vi "Get Sizes.vi"(2 "Array":variant) -> (0 "Sizes(s)":i32[](array[numeric]))   [LabVIEW 2019, in "Arrays.lvlib"]
uses:
  Arrays.lvlib
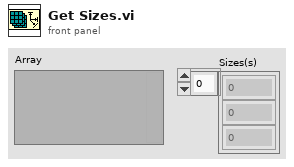
[diagram p1: front panel]
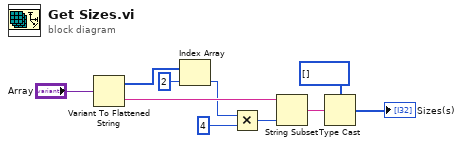
[diagram p0: block diagram]
diagram:
  n1 = Variant To Flattened String(Variant="Array") -> (data string=w7:string, 1:w10:i16[])
  n2 = Index Array(array=w10, index=2) -> (element=w2:i16)
  n3 = Multiply(x=w2, y=i16 4) -> (x*y=w6:i16)
  n4 = String Subset(string=w7, length (rest)=w6) -> (substring=w4:string)  [unwired: 1 in]
  n5 = Type Cast(type=i32[] [] ("value"), x=w4) -> (*(type *) &x=→"Sizes(s)":i32[])
